vi "FGV_PSP - Mercury Targets.vi"(4 "error in":errorcluster, 6 "Function":enum16{"write", "read"}(ring), 7 "Targets":T1) -> (0 "error out":errorcluster, 3 "Targets":T1)   [LabVIEW 2016]
uses:
  Typedefs/Targets.ctl
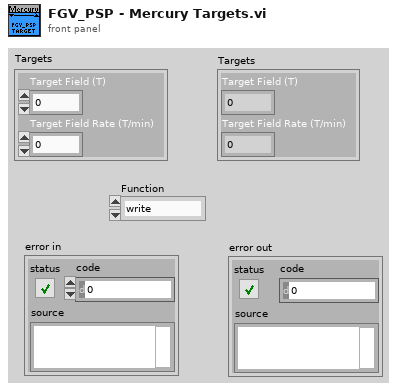
[diagram p1: front panel]
types:
  T1 = typedef "Targets.ctl" = cluster{"Target Field (T)":dbl, "Target Field Rate (T/min)":dbl}
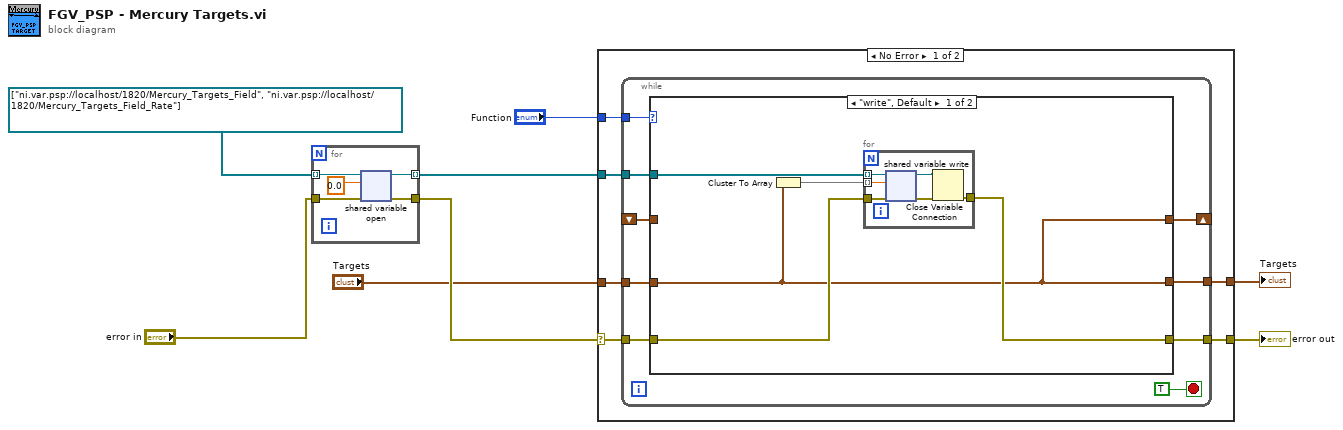
[diagram p0: block diagram]
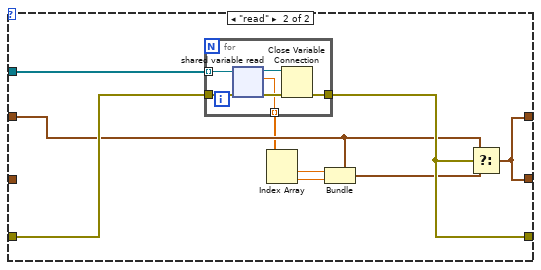
[diagram p2: hidden frame]
diagram:
  n1 = for {
    tunnel: [w13] -> w6 mode=indexing
    tunnel: [w12] -> w5
    tunnel: "error in" -> [w11]
    tunnel: refnum<k21>[] ["ni.var.psp://localhost/1820/Mercury_Targets_Field", "ni.var.psp://localhost/1820/Mercury_Targets_Field_Rate"] -> [w10] mode=indexing
    n2 = shared-variable-open(w10, w11, 0.0) -> (w13:refnum<k21>, w12:errorcluster)  [unwired: 1 in]
  }
  n3 = case shown="No Error" w5 {
    selector: w5 -> [w19 w56]
    tunnel: [w18 w56] -> w8
    tunnel: [w17 w55] -> w2
    tunnel: "Function" -> [w16 _]
    tunnel: w6 -> [w15 _]
    tunnel: "Targets" -> [w14 w55]
    frame No Error {
      n4 = while {
        shift-right: [w23] -> _
        shift-left: _ -> [w22]
        tunnel: w19 -> [w27]
        tunnel: [w26] -> w18
        tunnel: [w25] -> w17
        tunnel: w16 -> [w24]
        tunnel: w15 -> [w21]
        tunnel: w14 -> [w20]
        stop <- TRUE stop-if-true
        n5 = case shown="\"write\", Default" w24 {
          tunnel: w27 -> [w32 w46]
          tunnel: [w33 w45] -> w26
          tunnel: [w29 w48] -> w25
          tunnel: [w29 w48] -> w23
          tunnel: w22 -> [_ w44]
          tunnel: w21 -> [w31 w47]
          tunnel: w20 -> [w29 _]
          frame "write", Default {
            n6 = Cluster To Array(cluster=w29) -> (array=w30:dbl[])
            n7 = for {
              tunnel: [w38] -> w33
              tunnel: w32 -> [w36]
              tunnel: w31 -> [w35] mode=indexing
              tunnel: w30 -> [w34] mode=indexing
              n8 = shared-variable-write(w35, w36, w34) -> (w37:refnum<k21>, w39:errorcluster)
              n9 = Close Variable Connection(8:w39, 11:w37) -> (0:w38:errorcluster)
            }
          }
          frame "read" {
            n10 = for {
              tunnel: [w52] -> w45
              tunnel: w47 -> [w51] mode=indexing
              tunnel: w46 -> [w50]
              tunnel: [w49] -> w42 mode=indexing
              n11 = shared-variable-read(w51, w50) -> (w54:refnum<k21>, w53:errorcluster, w49:dbl)  [unwired: 1 out]
              n12 = Close Variable Connection(8:w53, 11:w54) -> (0:w52:errorcluster)
            }
            n13 = Index Array(array=w42) -> (element #1=w41:dbl, element #2=w40:dbl)  [unwired: 2 in]
            n14 = Bundle(cluster=w44, "Target Field (T)"=w41, "Target Field Rate (T/min)"=w40) -> (w43:T1)
            n15 = Select(t=w44, s=w45, f=w43) -> (s? t:f=w48:T1)
          }
        }
      }
    }
    frame Error {
    }
  }
  "error out" <- w8
  "Targets" <- w2
